vi "createNdimArray.vi"(0 "Array 1":dbl[](array[numeric])=[1.0, 1.0, 1.0, 1.0, 1.0, 1.0], 5 "Array 2":dbl[](array[numeric])=[2.0, 2.0, 2.0, 2.0, 2.0], 7 "Array 3":dbl[](array[numeric])=[3.0, 3.0, 3.0], 9 "Array 4":dbl[](array[numeric])=[4.0]) -> (4 "Output Array":dbl[][](array[numeric]), 6 "Number of Elements":i32, 8 "Number of Elements":i32, 10 "Number of Elements":i32, 15 "Number of Elements":i32)   [LabVIEW 2011]
doc: "HOW TO USE THIS EXAMPLE:\n\n1. Examine the arrays to the right. As you can see, there are four arrays, each with a \ndifferent number of elements. \n\n2. Run the VI. \n\n3. Now, you can see that the four arrays have been combined to create a 2-dimensional array that maintains the individual sub-array elements and array sizes. This type of data type could be useful in creating objects such as Pareto matrices. \n\nHOW TO CREATE A 2-DIMENSIONAL ARRAY OF DIFFERENT-SIZED SUB-ARRAYS:\n\n1. Create a sub-array by placing a digital control (Controls >> Numeric >> Digital Control) inside an empty array shell (Controls >> Array and Cluster >> Array).\n\n2. Place the numeric array that you created in Step 1 into an empty cluster shell (Controls >> Array and Cluster >> Cluster).\n\n3. Place the cluster of an array that you created in Step 2 into an empty array shell (Controls >> Array and Cluster >> Array).\n\n4. Now you can expand the array of clusters out to accommodate the various sub-arrays."
panel:
  out "Number of Elements":i32=3
  out "Number of Elements":i32=1
  out "Number of Elements":i32=5
  out "Number of Elements":i32=6
  # "How To Use This Example Program:"
  # "1. Examine the arrays to the right.  As you can see, there are four arrays, each with a different number of elements.  \n\n2. Run the VI.\n\n3. Now, you can see that the four arrays have been combined to create a 2-dimensional array that contains the individual sub-array elements and array sizes.  \n\nThis type of data could be useful in creating objects such as Pareto matrices.\n\n*Note: As you can see, the unused array elements will contain zeros.  As long as you use the first element of the array as a record of the sub-array size, you will maintain the integrity of the sub-array."
  # "Sub-Array 1"
  # "Sub-Array 2"
  # "Sub-Array 3"
  # "Sub-Array 4"
  # "Number of Elements in Sub-Arrays:"
  # "Elements in Sub-Arrays:"
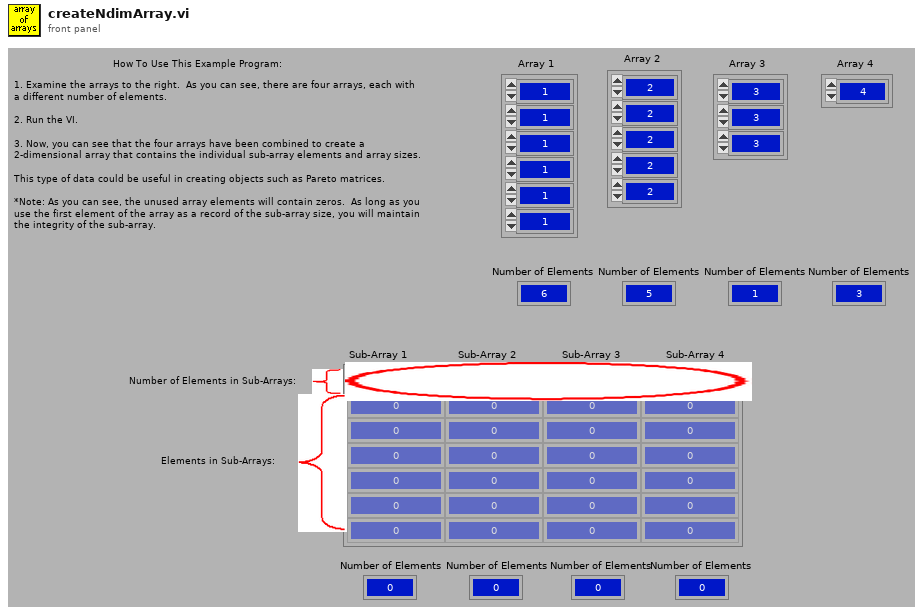
[diagram p1: front panel]
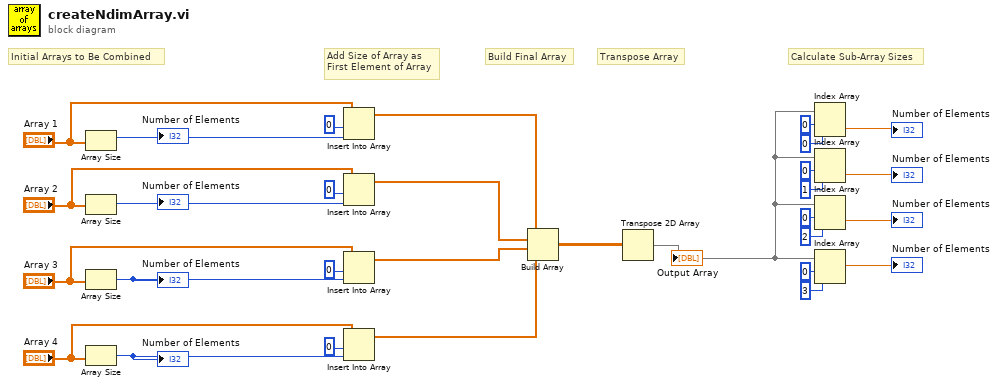
[diagram p0: block diagram]
diagram:
  # "Transpose Array"
  # "Add Size of Array as \nFirst Element of Array"
  # "Calculate Sub-Array Sizes"
  # "Build Final Array"
  # "Initial Arrays to Be Combined"
  n1 = Array Size(array="Array 1") -> (size(s)=w28:i32)
  "Number of Elements" <- w28
  n2 = Array Size(array="Array 2") -> (size(s)=w29:i32)
  "Number of Elements" <- w29
  n3 = Array Size(array="Array 3") -> (size(s)=w20:i32)
  "Number of Elements" <- w20
  n4 = Array Size(array="Array 4") -> (size(s)=w27:i32)
  "Number of Elements" <- w27
  n5 = Insert Into Array "Insert Into Array"(array="Array 1", index=0 ("Index"), new element=w28) -> (w24:dbl[])
  n6 = Insert Into Array "Insert Into Array"(array="Array 2", index=0 ("Index"), new element=w29) -> (w18:dbl[])
  n7 = Insert Into Array "Insert Into Array"(array="Array 3", index=0 ("Index"), new element=w20) -> (w15:dbl[])
  n8 = Insert Into Array "Insert Into Array"(array="Array 4", index=0 ("Index"), new element=w27) -> (w17:dbl[])
  n9 = Build Array "Build Array"(w24, w18, w15, w17) -> (w14:dbl[][])
  n10 = Transpose 2D Array(2D array=w14) -> (transposed array=w4:dbl[][])
  "Output Array" <- w4
  n11 = Index Array(array=w4, index (row)=0 ("Index (row)"), index (col)=0 ("Disabled Index (col)")) -> (element=→"Number of Elements":dbl)
  n12 = Index Array(array=w4, index (row)=0 ("Index (row)"), index (col)=1 ("Disabled Index (col)")) -> (element=→"Number of Elements":dbl)
  n13 = Index Array(array=w4, index (row)=0 ("Index (row)"), index (col)=2 ("Disabled Index (col)")) -> (element=→"Number of Elements":dbl)
  n14 = Index Array(array=w4, index (row)=0 ("Index (row)"), index (col)=3 ("Disabled Index (col)")) -> (element=→"Number of Elements":dbl)
